vi "Check Message.vi"(8 "error in (no error)":errorcluster, 9 "Echo Received":string, 10 "Message Sent":string, 11 "Actuator in":refnum<class "Actuator.lvclass">) -> (0 "error out":errorcluster, 2 "Command Sucessful?":bool, 3 "Actuator out":refnum<class "Actuator.lvclass">)   [LabVIEW 2021, in "Actuator.lvclass"]
uses:
  Actuator.lvclass
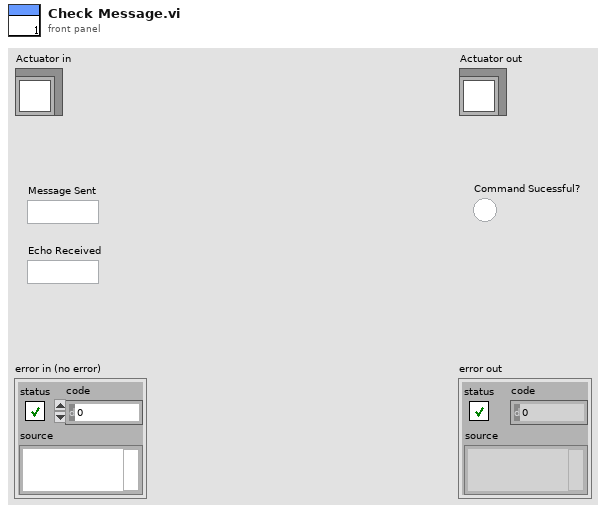
[diagram p1: front panel]
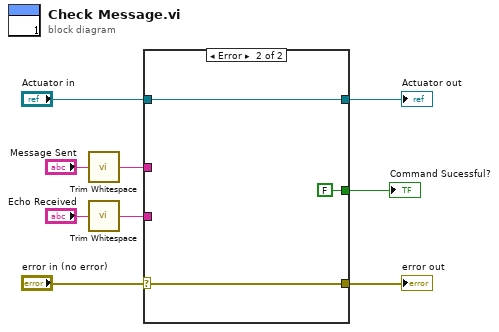
[diagram p0: block diagram]
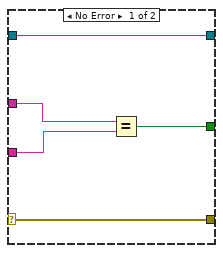
[diagram p2: hidden frame]
diagram:
  n1 = call <vilib>:"Trim Whitespace.vi"("string"="Message Sent") -> ("trimmed string"=w1:string)  [unwired: 1 in]
  n2 = call <vilib>:"Trim Whitespace.vi"("string"="Echo Received") -> ("trimmed string"=w2:string)  [unwired: 1 in]
  n3 = case shown="Error" "error in (no error)" {
    selector: "error in (no error)" -> [w13 w17]
    tunnel: [w13 w17] -> w8
    tunnel: [w14 w16] -> w6
    tunnel: "Actuator in" -> [w14 w16]
    tunnel: w1 -> [w12 _]
    tunnel: w2 -> [w11 _]
    tunnel: [w10 FALSE] -> w3
    frame No Error {
      n4 = Equal?(x=w12, y=w11) -> (x = y?=w10:bool)
    }
    frame Error {
    }
  }
  "error out" <- w8
  "Actuator out" <- w6
  "Command Sucessful?" <- w3
